vi "New QControl_Graph.vi"(11 "Reference":refnum<vi>) -> (0 "error out":errorcluster, 3 "QControl_Graph out":refnum<class "QControl_Graph.lvclass">, 5 "Action Performed":refnum<user-event>)   [LabVIEW 2017, in "QControl_Graph.lvclass"]
doc: "The Constructor Method is the method that instantiates the new QControl Class. It is named \"New\" and then the name of the QControl Class (i.e. New StatusHistory.vi). Its only input is the control reference that the new QControl Class will control. \n\nThe Constructor will then:\n1. Cast the reference to \"Generic\" and call the Load Reference Method to load the control reference to the class private data \n2. Call the Load State Data Method which loads the State Data DVR to the class private data\n3. Call the Initialize Method to perform any initialization and start any other references used by the QControl Class and launch the Event Handler\n\nThe output of the Constructor Method is the QControl Class Wire. This wire should be handled and passed just like the reference of a basic control/indicator. <b>Any manipulation of the control after the Constructor Method should use Properties or Methods on this wire or handle UI Logic in the Event Handler.</b>\n<b> </b> <b> </b>\n©2016 Q Software Innovations, LLC (QSI)\nwritten by Quentin Alldredge\nproduced in LabVIEW 2015\n\nsupport@qsoftwareinnovations.com\nwww.qsoftwareinnovations.com\n\nAll rights reserved.\n\nRedistribution and use in source and binary forms, with or without modification, are permitted provided that the following conditions are met:\n\n * Redistributions of source code must retain the above copyright notice, this list of conditions and the following disclaimer.\n * Redistributions in binary form must reproduce the above copyright notice, this list of conditions and the following disclaimer in the documentation and/or other materials provided with the distribution.\n * Neither the name of Q Software Innovations, LLC. nor the names of its contributors may be used to endorse or promote products derived from this software without specific prior written permission.\n\nTHIS SOFTWARE IS PROVIDED BY THE COPYRIGHT HOLDERS AND CONTRIBUTORS \"AS IS\" AND ANY EXPRESS OR IMPLIED WARRANTIES, INCLUDING, BUT NOT LIMITED TO, THE IMPLIED WARRANTIES OF MERCHANTABILITY AND FITNESS FOR A PARTICULAR PURPOSE ARE DISCLAIMED. IN NO EVENT SHALL THE COPYRIGHT OWNER OR CONTRIBUTORS BE LIABLE FOR ANY DIRECT, INDIRECT, INCIDENTAL, SPECIAL, EXEMPLARY, OR CONSEQUENTIAL DAMAGES (INCLUDING, BUT NOT LIMITED TO, PROCUREMENT OF SUBSTITUTE GOODS OR SERVICES; LOSS OF USE, DATA, OR PROFITS; OR BUSINESS INTERRUPTION) HOWEVER CAUSED AND ON ANY THEORY OF LIABILITY, WHETHER IN CONTRACT, STRICT LIABILITY, OR TORT (INCLUDING NEGLIGENCE OR OTHERWISE) ARISING IN ANY WAY OUT OF THE USE OF THIS SOFTWARE, EVEN IF ADVISED OF THE POSSIBILITY OF SUCH DAMAGE."
uses:
  QControl_Graph.lvclass
  Actions.ctl
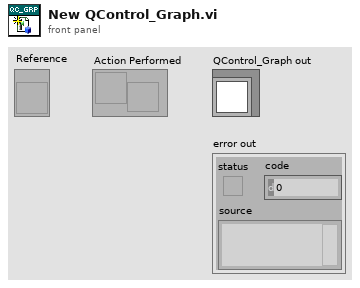
[diagram p1: front panel]
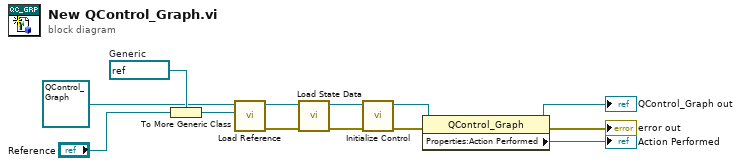
[diagram p0: block diagram]
diagram:
  w12 = refnum<vi> refnum  # Generic
  n1 = To More Generic Class(target class=w12, reference="Reference") -> (generic class reference=w13:refnum<vi>)
  n2 = call-dynamic "Load Reference.vi"("Reference"=w13, "QControl_Graph in"=refnum<class "QControl_Graph.lvclass"> refnum ("QControl_Graph.lvclass")) -> ("error out"=w9:errorcluster, "QControl_Graph out"=w7:refnum<class "QControl_Graph.lvclass">)  [unwired: 8 in]
  n3 = call-dynamic "Load State Data.vi"("error in (no error)"=w9, "QControl_Graph in"=w7) -> ("error out"=w8:errorcluster, "QControl_Graph out"=w6:refnum<class "QControl_Graph.lvclass">)  [unwired: 8 in]
  n4 = call-dynamic "Initialize Control.vi"("error in (no error)"=w8, "QControl_Graph in"=w6) -> ("error out"=w3:errorcluster, "QControl_Graph out"=w10:refnum<class "QControl_Graph.lvclass">)  [unwired: 8 in]
  n5 = property class="QControl_Graph"(reference=w10, error in=w3) -> (reference out=→"QControl_Graph out":refnum<class "QControl_Graph.lvclass">, error out=→"error out":errorcluster, "Properties:Action Performed"=→"Action Performed":refnum<user-event>)
